vi "Wave generator.vi"(10 "Timing Source":refnum<k21>="50MHz") -> (3 "Generated Data":i16)   [LabVIEW 2014]
uses:
  <vilib>/Platform/TimedLoop/XDataNode/timing_clust.ctl
  <vilib>/Platform/TimedLoop/XDataNode/nitl_modes.ctl
  <vilib>/Platform/TimedLoop/XDataNode/wakeup.ctl
  <vilib>/rvi/eio/common/nirviEmuTemplateMethod_errors.vi
  <vilib>/rvi/Emulation/niFpgaSctlEmulationGetInTimedLoop.vi
  <vilib>/rvi/Emulation/niFpgaEmulationReportErrorSimple.vi
  <vilib>/rvi/Emulation/niFpgaGetClockAttributes.vi
  <vilib>/rvi/Emulation/niFpgaCriticalErrorInLSC.vi
  <vilib>/rvi/Memory/Memory_Emulation/nirvimemoryEmulation.vi
  <vilib>/rvi/Memory/Memory_Emulation/nirvimemoryFastEmulation.vi
  <vilib>/rvi/DataTransferAndStorage/Container/Common/niFpgaContainerGetUniqueNameForEmu.vi
  <vilib>/rvi/Memory/Memory_Emulation/niFpgaMemoryEmulationCacheClearOnFirstRun.vi
  <vilib>/rvi/Memory/Memory_Emulation/nirvimemoryEmulationManagerCache_MakeExclusive.vi
  <vilib>/rvi/Memory/Memory_Emulation/niFpgaMemoryEmulationValidateCache.vi
  <vilib>/rvi/Memory/Memory_Emulation/nirvimemoryEmulationManagerCache_InsertValue.vi
  <vilib>/Utility/error.llb/Clear Errors.vi
  <vilib>/rvi/Memory/Memory_Emulation/nirvimemoryEmulationManagerCache_ReleaseExclusive.vi
  <vilib>/rvi/Memory/Memory_Emulation/nirvimemoryEmulationManagerCache_GetValue.vi
  <vilib>/rvi/Emulation/niFpgaEmulationIsFPGAContextNoSignature.vi
  <vilib>/rvi/Memory/Memory_Emulation/nirvimemoryEmulationManagerCache_SetValue.vi
  <vilib>/rvi/Emulation/niFpgaSctlEmulationResourceMgr.vi
  <vilib>/Platform/TimedLoop/XDataNode/XDataNode.xnode
  <vilib>/eio/EIOMethodNode/EIOMethodNode.xnode
  <vilib>/rvi/DataTransferAndStorage/Container/XNode/niFpgaContainer.xnode
  <vilib>/Platform/TimedLoop/XDataNode/XDNodeRunTimeDep.lvlib
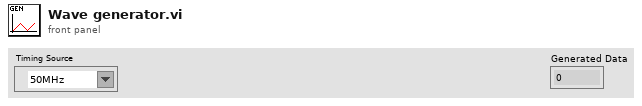
[diagram p1: front panel]
types:
  T1 = typedef "XDNodeRunTimeDep.lvlib/timing_clust.ctl" = cluster{"Expected End [f-1]":u64, "Actual End [f-1]":u64, "Finished Late? [f-1]":bool, "Expected End [i-1]":u64, "Actual End [i-1]":u64, "Finished Late? [i-1]":bool, "Expected Start [i]":u64, "Actual Start [i]":u64, "Expected Start [f]":u64, "Actual Start [f]":u64, "Source Name":string, "Structure Name":string, "Period":i64, "Deadline":i64, "Offset":i64, "Start":i64, "Priority":i32, "Timeout":i32, "Mode":T2, "Wakeup Reason":T3, "Error":errorcluster, "Source Type":string, "Secondary Source Type":string, "Global End Time":u64, "Global Start Time":u64, "Frame Duration":u64, "Iteration Duration":u64, "Assigned CPU":i32, "I/O Scan Engine Mode":u32}
  T2 = typedef "XDNodeRunTimeDep.lvlib/nitl_modes.ctl" = enum32{"No Change", "Process missed periods, maintain original phase", "Discard missed periods, maintain original phase", "Process missed periods, ignore original phase", "Discard missed periods, ignore original phase"}
  T3 = typedef "XDNodeRunTimeDep.lvlib/wakeup.ctl" = enum32{"Normal", "Aborted", "Asynchronous wakeup", "Timing source error", "Timed loop error", "Timeout"}
  T4 = cluster{"Boolean array[0]":bool, "Boolean array[1]":bool, "Boolean array[2]":bool, "Boolean array[3]":bool, "Boolean array[4]":bool, "Boolean array[5]":bool, "Boolean array[6]":bool, "Boolean array[7]":bool, "Boolean array[8]":bool, "Boolean array[9]":bool, "Boolean array[10]":bool, "Boolean array[11]":bool}
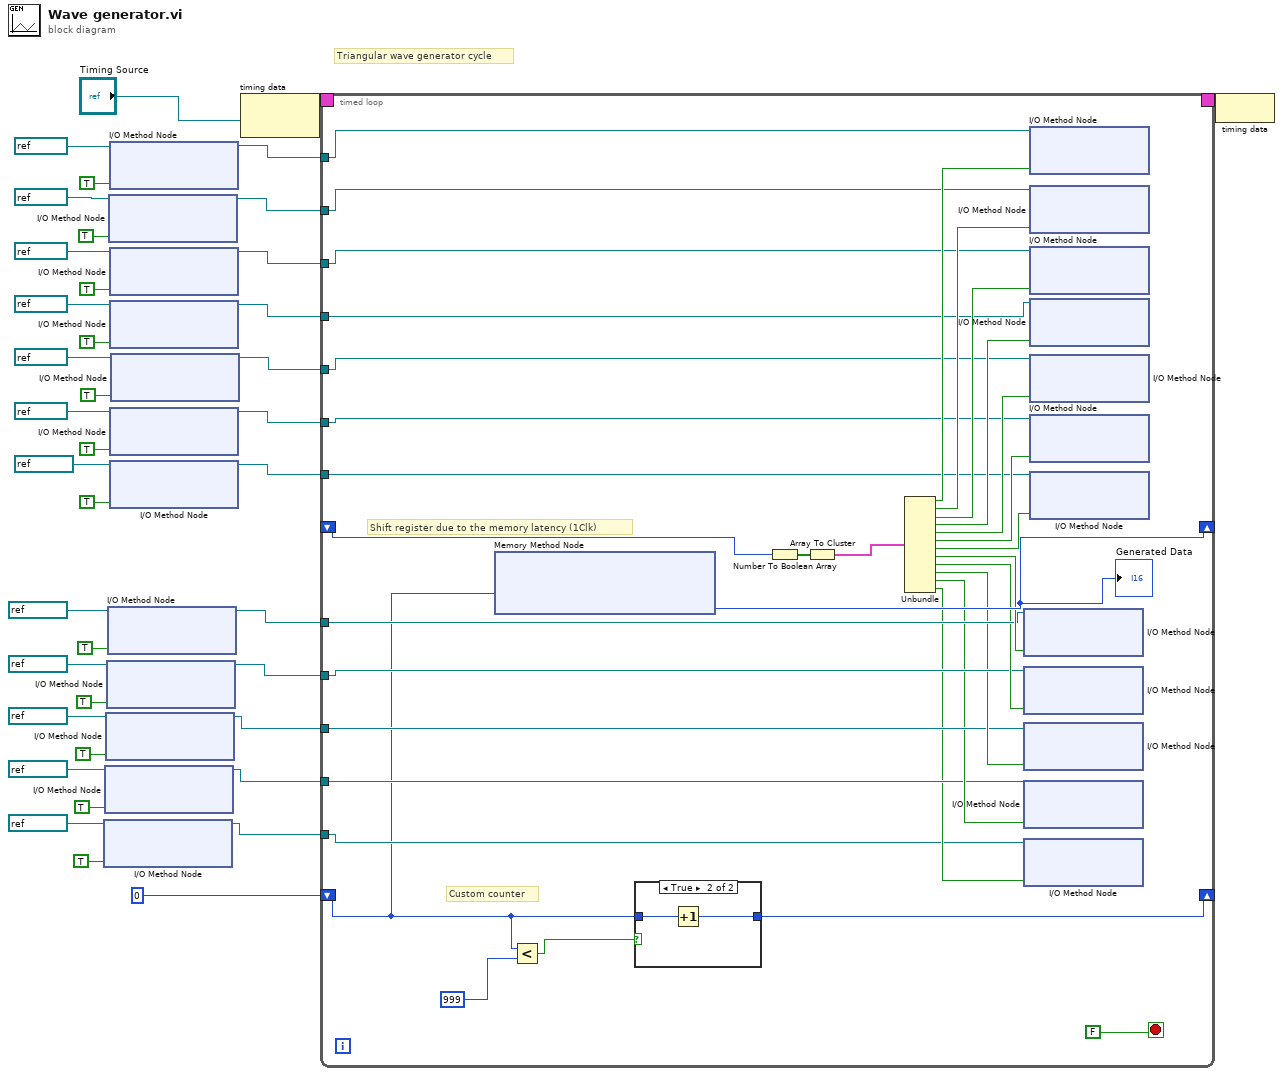
[diagram p0: block diagram]
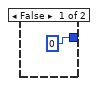
[diagram p2: hidden frame]
diagram:
  # "Triangular wave generator cycle"
  n1 = xnode "I/O Method Node"("FPGA I/O In"=refnum<k21> "DIO15", "Enable"=TRUE) -> ("FPGA I/O Out"=w3:refnum<k21>)
  n2 = xnode "I/O Method Node"("FPGA I/O In"=refnum<k21> "DIO14", "Enable"=TRUE) -> ("FPGA I/O Out"=w6:refnum<k21>)
  n3 = xnode "I/O Method Node"("FPGA I/O In"=refnum<k21> "DIO13", "Enable"=TRUE) -> ("FPGA I/O Out"=w9:refnum<k21>)
  n4 = xnode "I/O Method Node"("FPGA I/O In"=refnum<k21> "DIO12", "Enable"=TRUE) -> ("FPGA I/O Out"=w12:refnum<k21>)
  n5 = xnode "I/O Method Node"("FPGA I/O In"=refnum<k21> "DIO11", "Enable"=TRUE) -> ("FPGA I/O Out"=w15:refnum<k21>)
  n6 = xnode "I/O Method Node"("FPGA I/O In"=refnum<k21> "DIO5", "Enable"=TRUE) -> ("FPGA I/O Out"=w33:refnum<k21>)
  n7 = xnode "I/O Method Node"("FPGA I/O In"=refnum<k21> "DIO4", "Enable"=TRUE) -> ("FPGA I/O Out"=w36:refnum<k21>)
  n8 = xnode "I/O Method Node"("FPGA I/O In"=refnum<k21> "DIO6", "Enable"=TRUE) -> ("FPGA I/O Out"=w30:refnum<k21>)
  n9 = xnode "I/O Method Node"("FPGA I/O In"=refnum<k21> "DIO7", "Enable"=TRUE) -> ("FPGA I/O Out"=w27:refnum<k21>)
  n10 = xnode "I/O Method Node"("FPGA I/O In"=refnum<k21> "DIO9", "Enable"=TRUE) -> ("FPGA I/O Out"=w21:refnum<k21>)
  n11 = xnode "I/O Method Node"("FPGA I/O In"=refnum<k21> "DIO10", "Enable"=TRUE) -> ("FPGA I/O Out"=w18:refnum<k21>)
  n12 = xnode "I/O Method Node"("FPGA I/O In"=refnum<k21> "DIO8", "Enable"=TRUE) -> ("FPGA I/O Out"=w24:refnum<k21>)
  n13 = node-c288("Timing Source") -> (w40:T1)
  n14 = timed-loop {
    timing: w40 -> [_]
    timing-out: [_] -> w39
    shift-right: [w72] -> _
    shift-left: u32 0 -> [w41]
    tunnel: w36 -> [w66]
    tunnel: w33 -> [w64]
    tunnel: w30 -> [w62]
    tunnel: w27 -> [w60]
    tunnel: w24 -> [w58]
    tunnel: w21 -> [w56]
    tunnel: w18 -> [w54]
    tunnel: w15 -> [w52]
    tunnel: w12 -> [w50]
    tunnel: w9 -> [w48]
    tunnel: w6 -> [w46]
    tunnel: w3 -> [w44]
    shift-right: [w69] -> _
    shift-left: _ -> [w68]
    stop <- FALSE stop-if-true
    # "Shift register due to the memory latency (1Clk)"
    # "Custom counter"
    n15 = xnode ("Memory Method Node")("Address"=w41) -> ("Data"=w69:i16)  [unwired: 1 in, 1 out]
    "Generated Data" <- w69
    n16 = Less?(x=w41, y=u32 999) -> (x < y?=w42:bool)
    n17 = case shown="True" w42 {
      tunnel: w41 -> [_ w76]
      tunnel: [u32 0 w75] -> w72
      frame False {
      }
      frame True {
        n18 = Increment(x=w76) -> (x+1=w75:u32)
      }
    }
    n19 = Number To Boolean Array(number=w68) -> (Boolean array=w71:bool[])
    n20 = Array To Cluster(array=w71) -> (cluster=w70:T4)
    n21 = Unbundle(w70) -> ("Boolean array[0]"=w67:bool, "Boolean array[1]"=w65:bool, "Boolean array[2]"=w63:bool, "Boolean array[3]"=w61:bool, "Boolean array[4]"=w59:bool, "Boolean array[5]"=w57:bool, "Boolean array[6]"=w55:bool, "Boolean array[7]"=w53:bool, "Boolean array[8]"=w51:bool, "Boolean array[9]"=w49:bool, "Boolean array[10]"=w47:bool, "Boolean array[11]"=w45:bool)
    n22 = xnode "I/O Method Node"("FPGA I/O In"=w52, "Data"=w53) -> ()  [unwired: 1 out]
    n23 = xnode "I/O Method Node"("FPGA I/O In"=w50, "Data"=w51) -> ()  [unwired: 1 out]
    n24 = xnode "I/O Method Node"("FPGA I/O In"=w48, "Data"=w49) -> ()  [unwired: 1 out]
    n25 = xnode "I/O Method Node"("FPGA I/O In"=w46, "Data"=w47) -> ()  [unwired: 1 out]
    n26 = xnode "I/O Method Node"("FPGA I/O In"=w44, "Data"=w45) -> ()  [unwired: 1 out]
    n27 = xnode "I/O Method Node"("FPGA I/O In"=w66, "Data"=w67) -> ()  [unwired: 1 out]
    n28 = xnode "I/O Method Node"("FPGA I/O In"=w64, "Data"=w65) -> ()  [unwired: 1 out]
    n29 = xnode "I/O Method Node"("FPGA I/O In"=w62, "Data"=w63) -> ()  [unwired: 1 out]
    n30 = xnode "I/O Method Node"("FPGA I/O In"=w60, "Data"=w61) -> ()  [unwired: 1 out]
    n31 = xnode "I/O Method Node"("FPGA I/O In"=w58, "Data"=w59) -> ()  [unwired: 1 out]
    n32 = xnode "I/O Method Node"("FPGA I/O In"=w56, "Data"=w57) -> ()  [unwired: 1 out]
    n33 = xnode "I/O Method Node"("FPGA I/O In"=w54, "Data"=w55) -> ()  [unwired: 1 out]
  }
  n34 = node-c288(w39) -> ()
